vi "Simple_Example.vi"() -> ()   [LabVIEW 2024]
panel:
  out "text":string
  in  "file (use dialog)":path
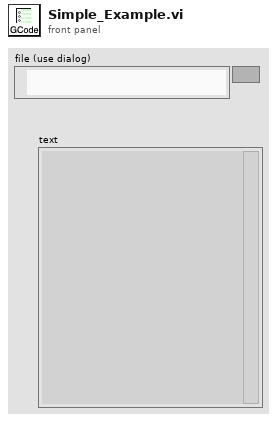
[diagram p1: front panel]
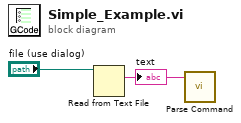
[diagram p0: block diagram]
diagram:
  n1 = Read from Text File(file (use dialog)="file (use dialog)") -> (text=w1:string)  [unwired: 3 in, 3 out]
  "text" <- w1
  n2 = call <userlib>:"Parse Command.vi"("text"=w1) -> ()  [unwired: 8 in, 3 out]
